vi "_Input Name to CSM Mode.vi"(11 "String":string) -> (1 "Queue Name":string, 2 "CSM Mode":T1, 3 "String(dup)":string)   [LabVIEW 2014, in "Communicable State Machine.lvlib"]
uses:
  Communicable State Machine.lvlib
  Typedef/_CSM_MODE.ctl
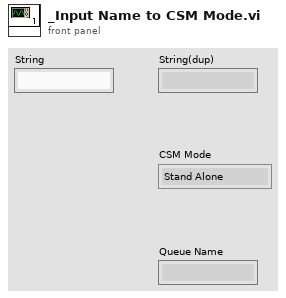
[diagram p1: front panel]
types:
  T1 = typedef "Communicable State Machine.lvlib/_CSM_MODE.ctl" = enum16{"Stand Alone", "CSM", "Action Worker"}
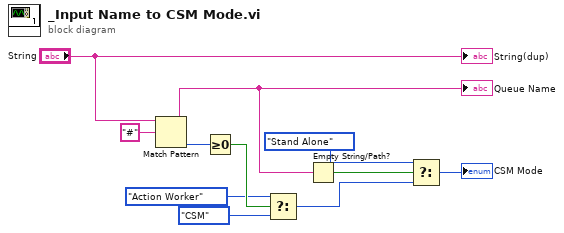
[diagram p0: block diagram]
diagram:
  n1 = Match Pattern(string="String", regular expression="#") -> (before substring=w3:string, offset past match=w9:i32)  [unwired: 1 in, 2 out]
  "Queue Name" <- w3
  n2 = Greater Or Equal To 0?(x=w9) -> (x >= 0?=w8:bool)
  n3 = Select(t=_CSM_MODE."Action Worker" ("Mode"), s=w8, f=_CSM_MODE."CSM" ("Mode")) -> (s? t:f=w4:T1)
  n4 = Empty String/Path?(string/path=w3) -> (empty?=w1:bool)
  n5 = Select(t=_CSM_MODE."Stand Alone" ("Mode"), s=w1, f=w4) -> (s? t:f=→"CSM Mode":T1)
  "String(dup)" <- "String"
